vi "Database.vi"(8 "error in (no error)":errorcluster) -> (0 "error out":errorcluster)   [LabVIEW 2017]
uses:
  Type Definitions/Queue FG Options.ctl
  Type Definitions/DB Data.ctl
  Type Definitions/DB Info.ctl
  Type Definitions/Controller Message.ctl
  Type Definitions/Controller States.ctl
  Type Definitions/Controller Data.ctl
  Type Definitions/Display Data.ctl
  Type Definitions/DB Record.ctl
  Type Definitions/Display Console States.ctl
  Type Definitions/GUI Data.ctl
  Type Definitions/Sensor UI Data.ctl
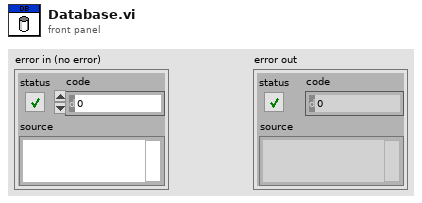
[diagram p1: front panel]
types:
  T1 = typedef "Queue FG Options.ctl" = enum16{"Set", "Get", "Read", "Write", "Destroy"}
  T2 = typedef "DB Data.ctl" = cluster{"Account":i32, "First Name":string, "Last Name":string, "Balance":fxp<+/-,64,35>, "DB Info":T3}
  T3 = typedef "DB Info.ctl" = enum16{"Empty", "Verify", "Login Accepted", "Invalid Login", "Deposit Complete", "Withdrawal Complete", "Withdrawal Failed", "Terminate"}
  T4 = typedef "Controller States.ctl" = enum16{"Timeout", "Initial", "Login", "Idle", "Balance Inquiry", "Deposit", "Withdrawal", "Fast Cash", "Terminate", "Wait on Exit", "Shutdown", "Error Handler"}
  T5 = typedef "Controller Data.ctl" = cluster{"Time":dbl, "DB Data in":T2, "Display Data":T6, "GUI Data ":T9, "Sensor UI":T10, "Controller States":T4}
  T6 = typedef "Display Data.ctl" = cluster{"Message Text":string, "DB Record":T7, "Card Read":bool, "Display Console States":T8}
  T7 = typedef "DB Record.ctl" = cluster{"Account":i32, "First Name":string, "Last Name":string, "Balance":fxp<+/-,64,35>}
  T8 = typedef "Display Console States.ctl" = enum16{"Timeout", "Initial", "Login", "Invalid Login", "Idle", "Balance Inquiry", "Deposit", "Withdrawal", "Fast Cash", "Withdrawal Failed", "Withdrawal Complete", "Terminate", "Shutdown"}
  T9 = typedef "GUI Data.ctl" = cluster{"Card Reader":enum8{"Enabled", "Disabled", "Disabled and Grayed Out"}, "Keypad":enum8{"Enabled", "Disabled", "Disabled and Grayed Out"}, "Balance Inquiry":enum8{"Enabled", "Disabled", "Disabled and Grayed Out"}, "Deposit":enum8{"Enabled", "Disabled", "Disabled and Grayed Out"}, "Withdrawal":enum8{"Enabled", "Disabled", "Disabled and Grayed Out"}, "Fast Cash":enum8{"Enabled", "Disabled", "Disabled and Grayed Out"}, "New Transaction":enum8{"Enabled", "Disabled", "Disabled and Grayed Out"}, "Terminate Session":enum8{"Enabled", "Disabled", "Disabled and Grayed Out"}, "Pinpad Value":string, "Timeout":i32, "Controller States":T4}
  T10 = typedef "Sensor UI Data.ctl" = cluster{"Funds dispensed":enum16{"Enabled", "Disabled", "Disabled and Grayed Out"}, "Deposit received":enum16{"Enabled", "Disabled", "Disabled and Grayed Out"}, "Timeout":dbl}
  T11 = typedef "Controller Message.ctl" = cluster{"Message Info":T4, "Message Data":variant}
  T12 = typedef "Database Message.ctl" = cluster{"Message Info":T13, "Message Data":variant}
  T13 = typedef "Database States.ctl" = enum16{"Initial", "Verify", "Balance Inquiry", "Deposit", "Withdrawal", "Fast Cash", "Terminate", "Shutdown"}
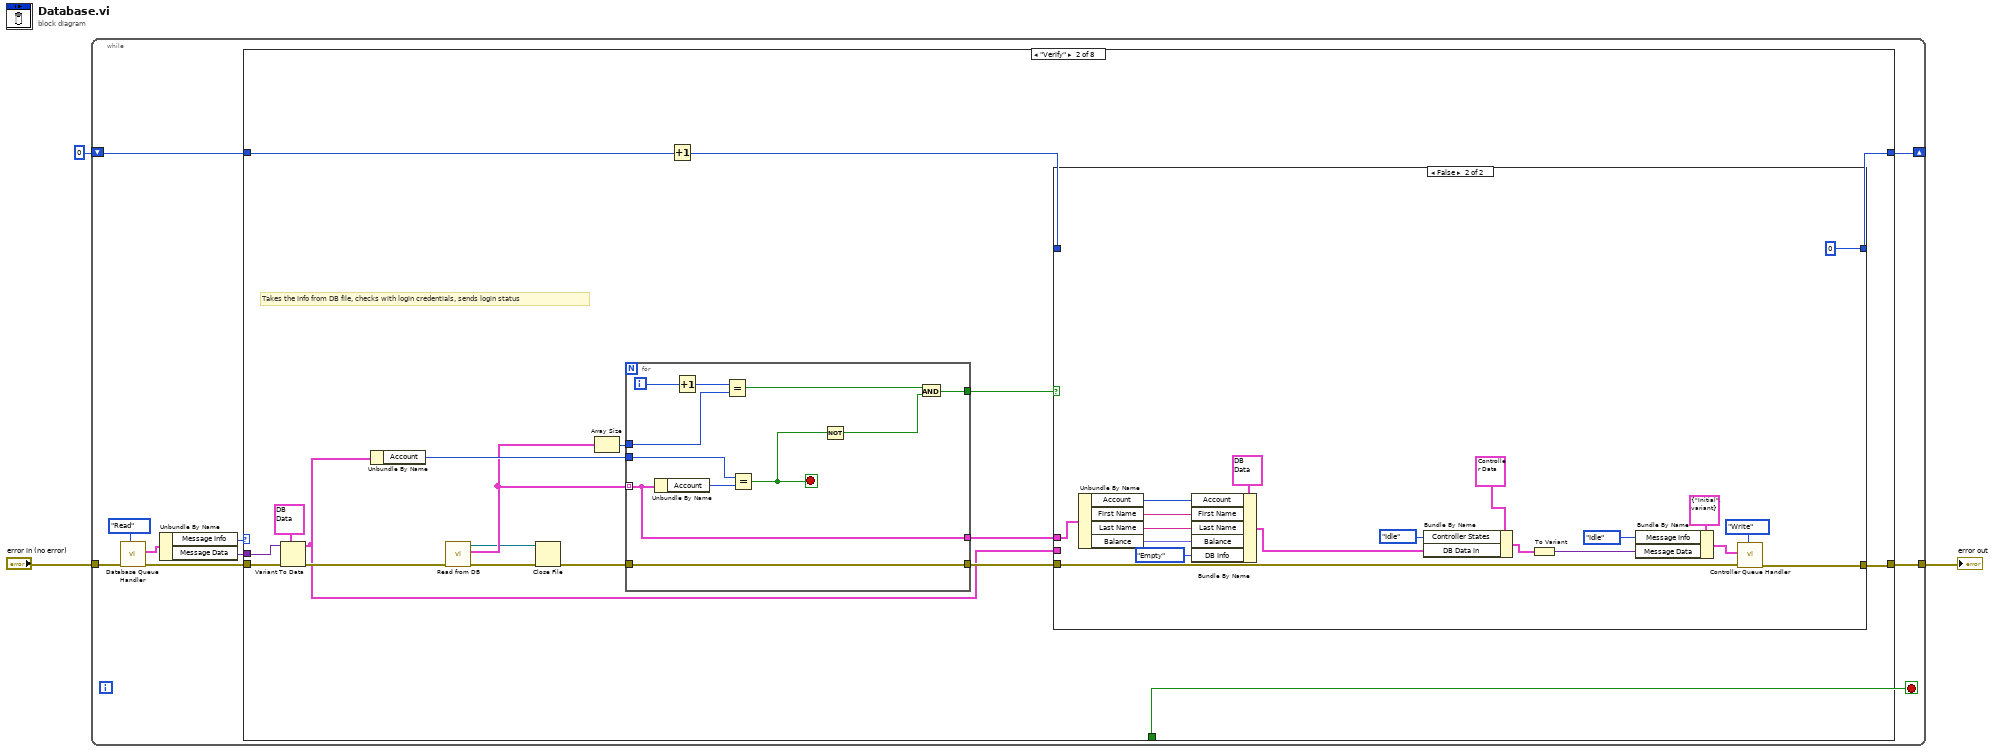
[diagram p0: block diagram]
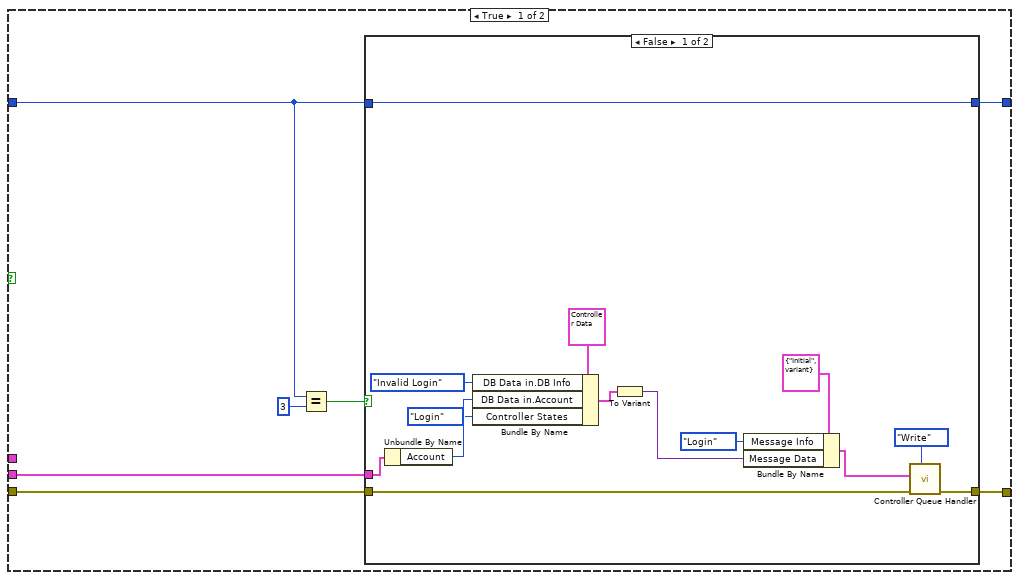
[diagram p3: hidden frame]
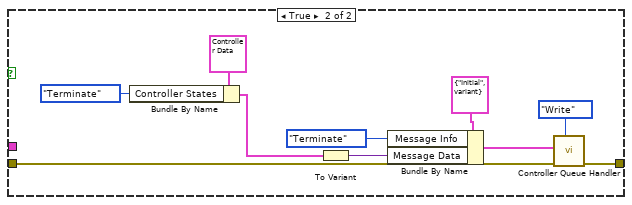
[diagram p4: hidden frame]
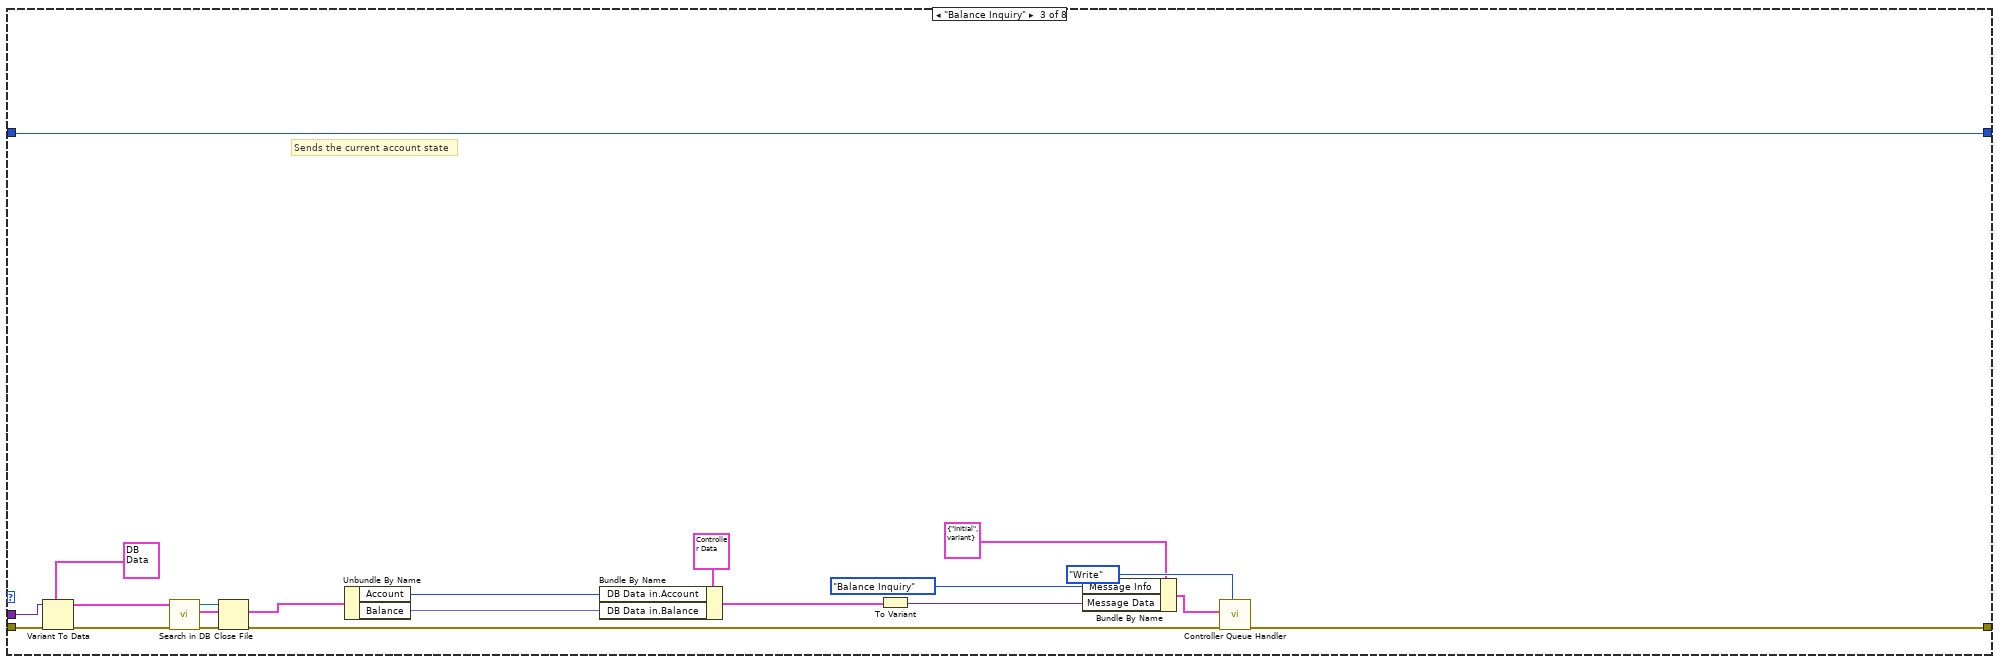
[diagram p5: hidden frame]
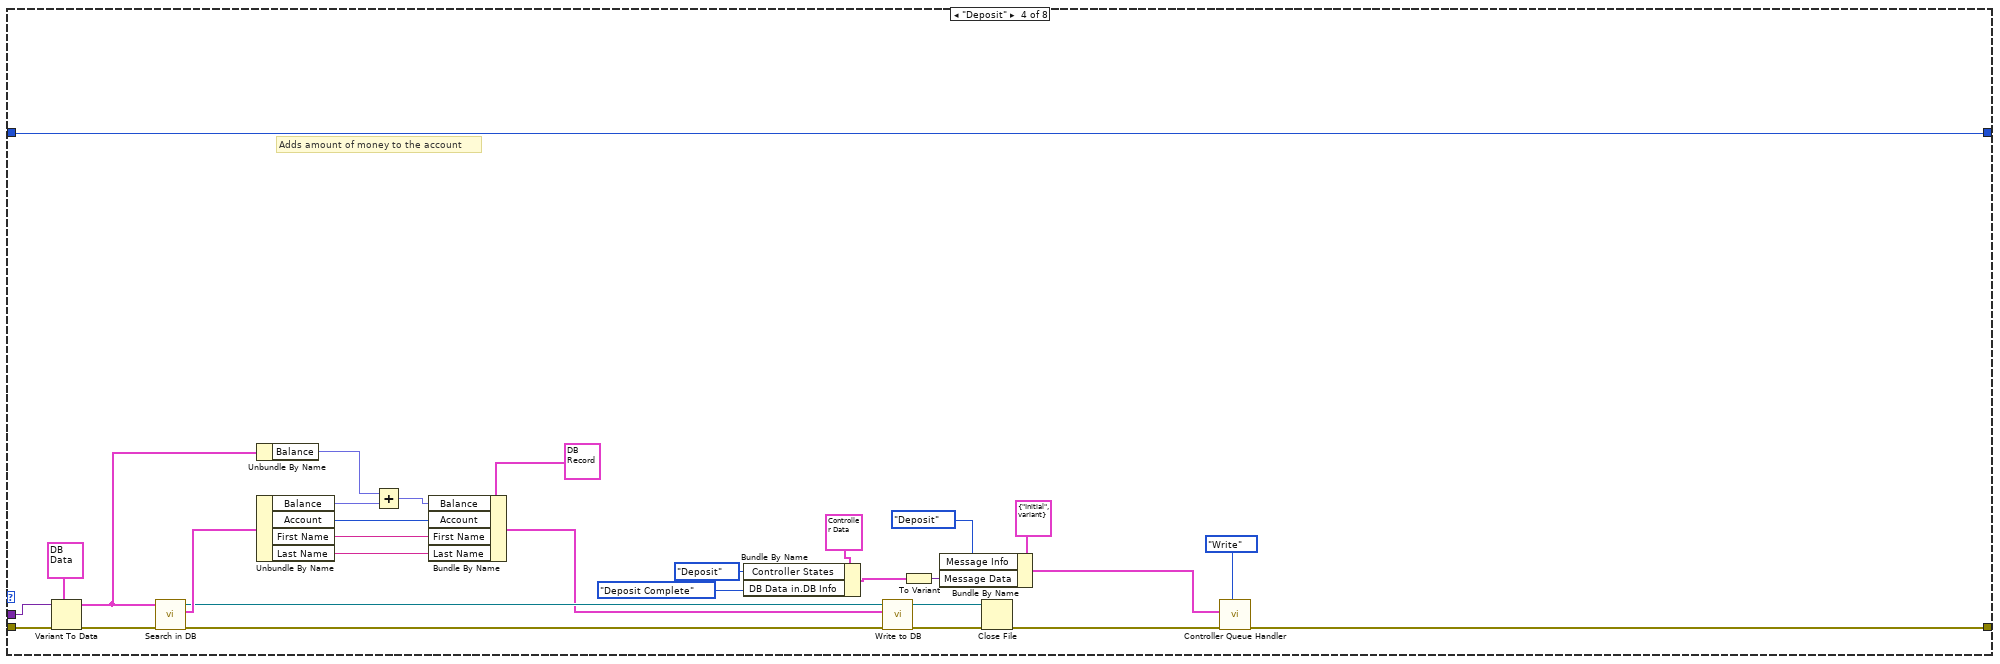
[diagram p6: hidden frame]
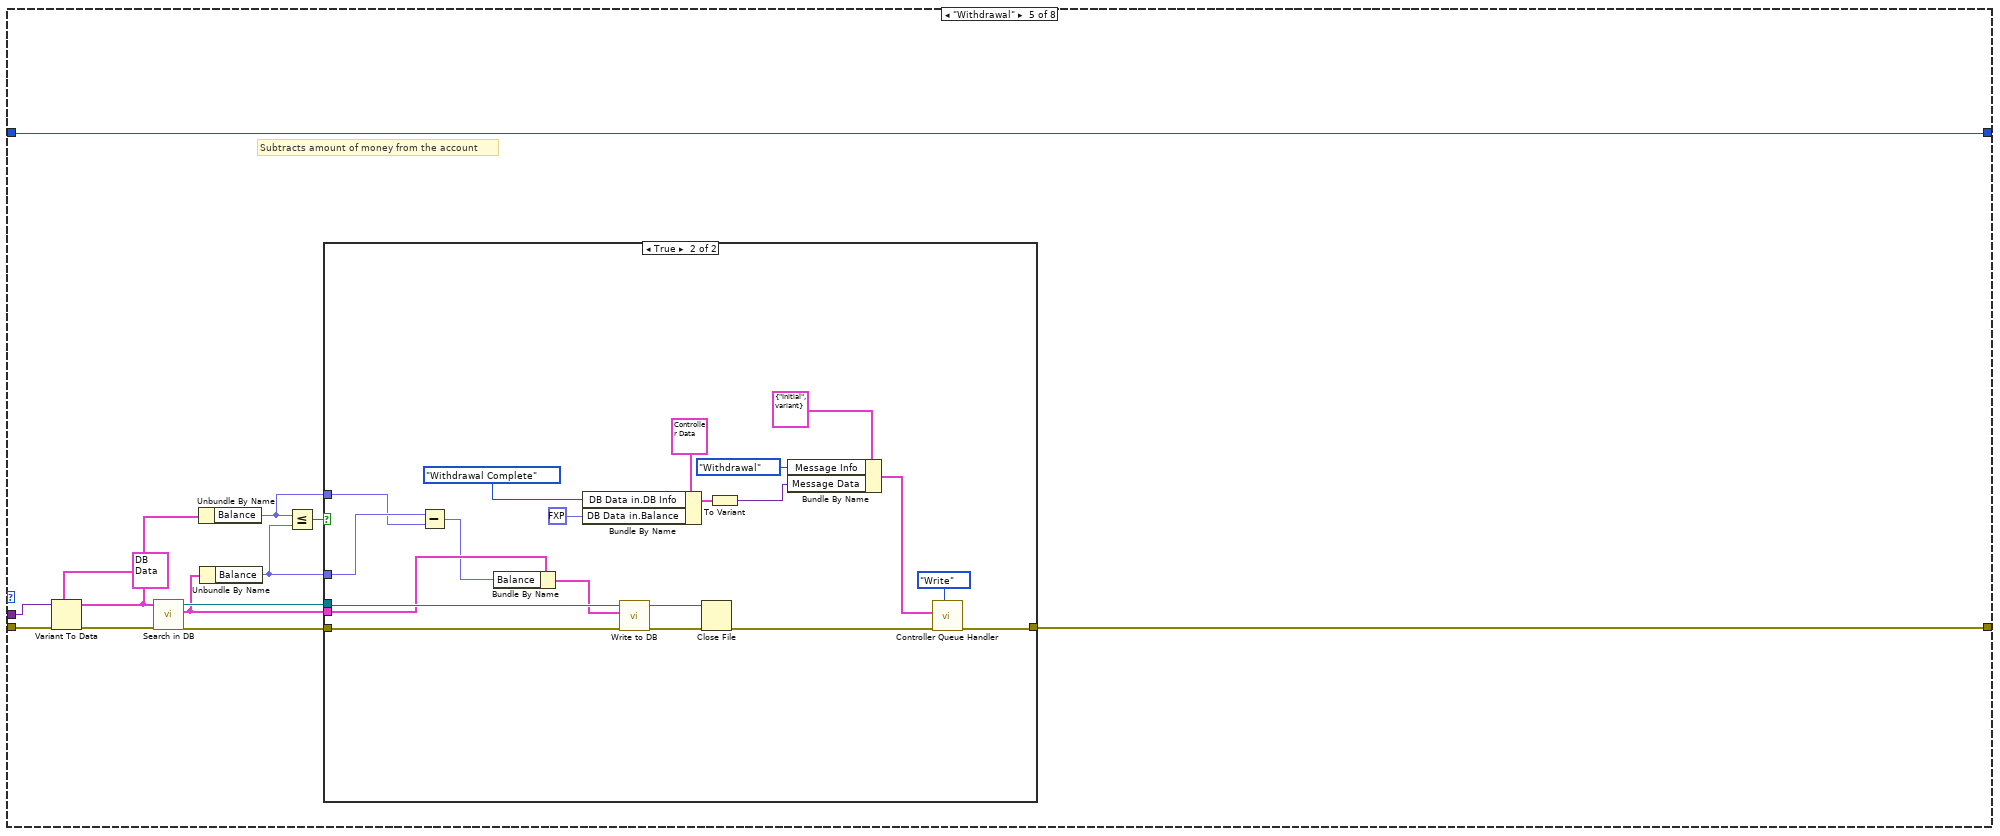
[diagram p7: hidden frame]
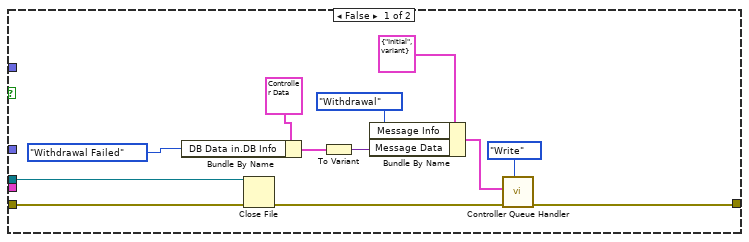
[diagram p8: hidden frame]
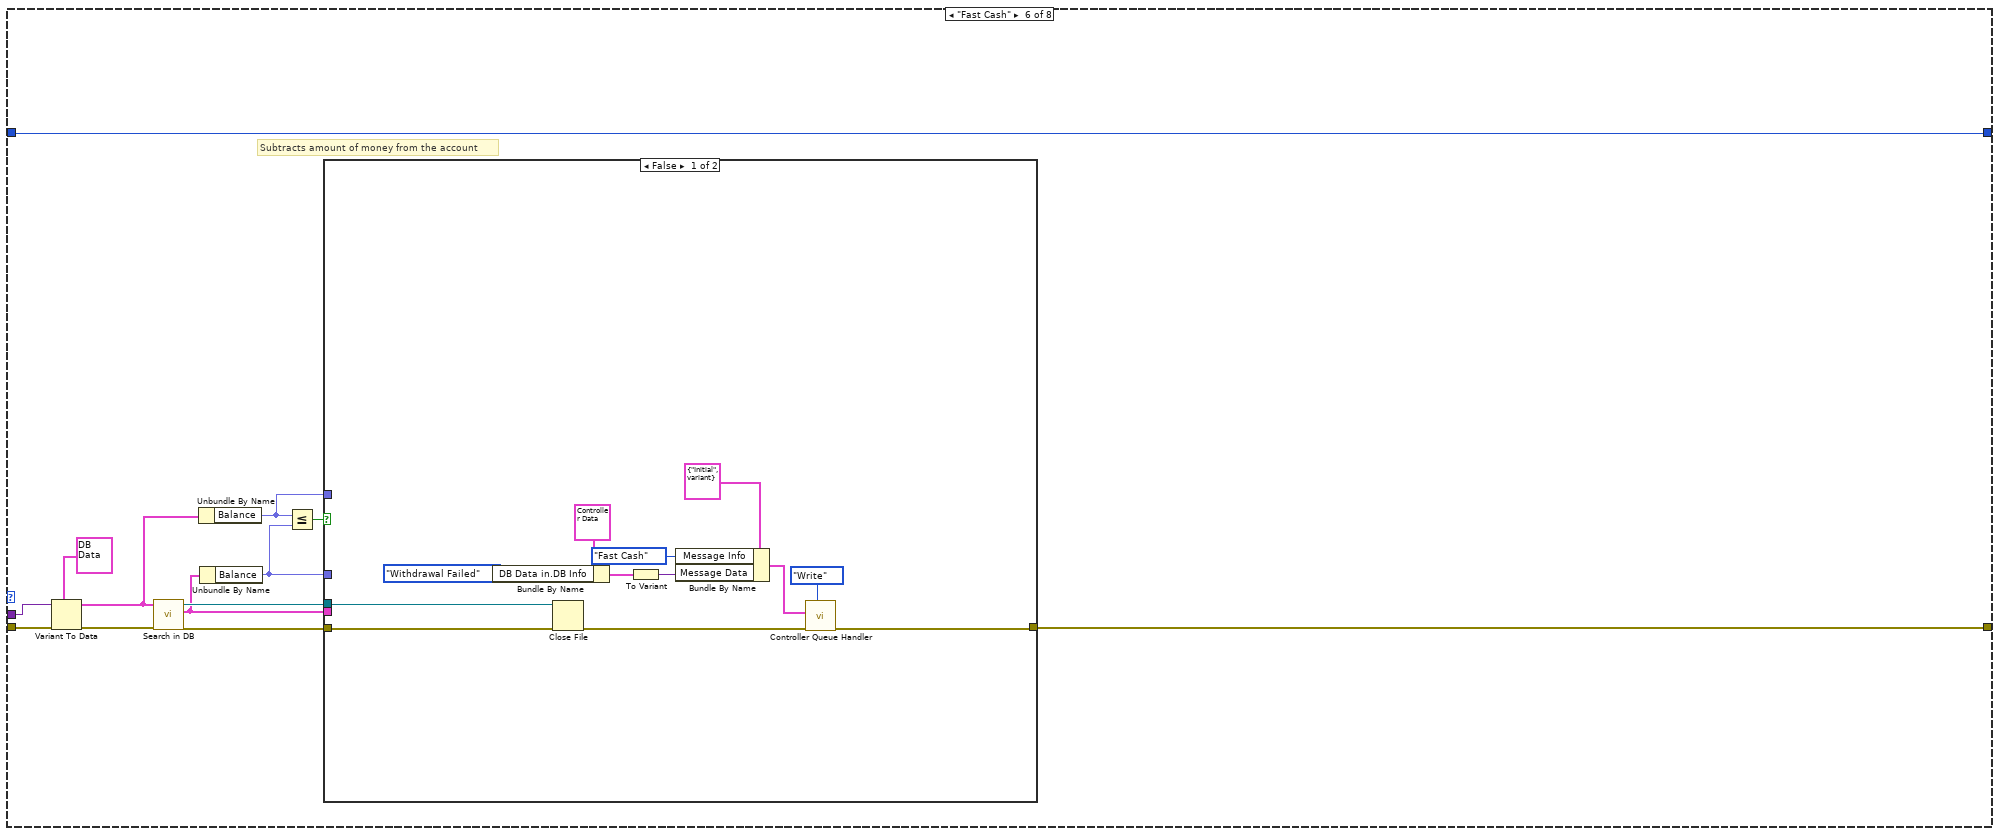
[diagram p9: hidden frame]
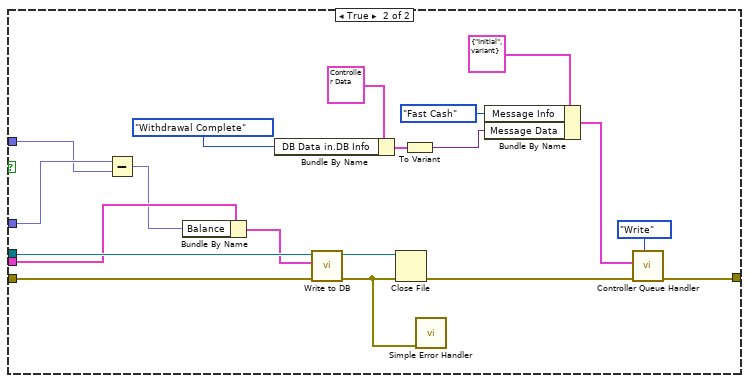
[diagram p10: hidden frame]
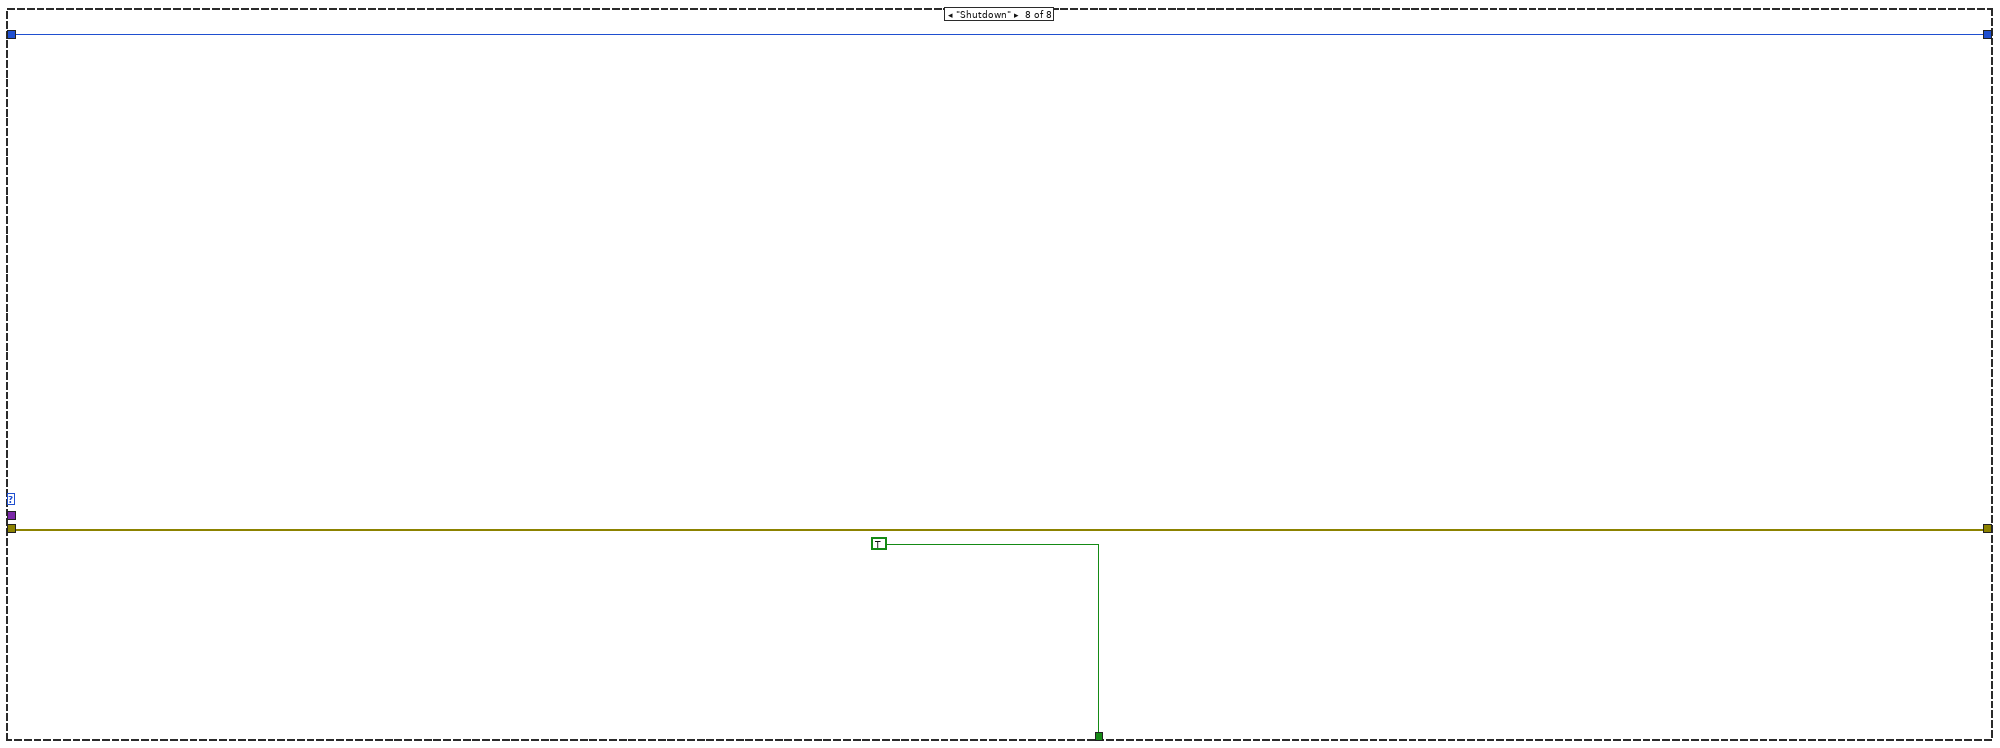
[diagram p12: hidden frame]
diagram:
  n1 = while {
    tunnel: "error in (no error)" -> [w12]
    tunnel: [w7] -> w2
    shift-right: [w5] -> _
    shift-left: 0 -> [w4]
    stop <- w6 stop-if-true
    n2 = call "Database Queue Handler.vi"("Action"=Queue_FG_Options."Read", "error in (no error)"=w12) -> ("error out"=w8:errorcluster, "Message out"=w11:T12)  [unwired: 7 in, 1 out]
    n3 = Unbundle By Name(w11) -> ("Message Info"=w10:T13, "Message Data"=w9:variant)
    n4 = case shown="\"Verify\"" w10 {
      tunnel: w9 -> [_ w31 w111 w141 w154 w199 _ _]
      tunnel: w8 -> [w15 w33 w114 w144 w157 w202 w235 w238]
      tunnel: [w15 w18 w108 w126 w148 w193 w235 w238] -> w7
      tunnel: [_ _ _ _ _ _ _ TRUE] -> w6
      tunnel: [w14 w17 w113 w143 w156 w201 w234 w236] -> w5
      tunnel: w4 -> [w14 w25 w113 w143 w156 w201 w234 w236]
      frame "Initial", Default {
      }
      frame "Verify" {
        # "Takes the info from DB file, checks with login credentials, sends login status"
        n5 = Variant To Data(error in=w33, type=T2 {"Account"=0, "First Name"="", "Last Name"="", "Balance"=0.0, "DB Info"=enum."Login Accepted"} ("DB Data in"), Variant=w31) -> (data=w20:T2, error out=w32:errorcluster)
        n6 = Unbundle By Name(w20) -> ("Account"=w29:i32)
        n7 = call "Read from DB.vi"("error in (no error)"=w32) -> ("error out"=w28:errorcluster, "Array"=w23:T7[], "refnum out"=w21:refnum<file>)  [unwired: 8 in]
        n8 = Close File(refnum=w21, error in=w28) -> (error out=w22:errorcluster)  [unwired: 1 out]
        n9 = Array Size(array=w23) -> (size(s)=w27:i32)
        n10 = for {
          tunnel: w29 -> [w43]
          tunnel: w23 -> [w34] mode=indexing
          tunnel: w22 -> [w35]
          tunnel: [w35] -> w24
          tunnel: w27 -> [w40]
          tunnel: [w36] -> w26
          tunnel: [w34] -> w16
          i -> [w42]
          stop <- w39 stop-if-true
          n11 = Unbundle By Name(w34) -> ("Account"=w44:i32)
          n12 = Increment(x=w42) -> (x+1=w41:i32)
          n13 = Equal?(x=w41, y=w40) -> (x = y?=w37:bool)
          n14 = Equal?(x=w43, y=w44) -> (x = y?=w39:bool)
          n15 = Not(x=w39) -> (.not. x?=w38:bool)
          n16 = And(x=w37, y=w38) -> (x .and. y?=w36:bool)
        }
        n17 = Increment(x=w25) -> (x+1=w19:i32)
        n18 = case shown="False" w26 {
          tunnel: w19 -> [w51 _]
          tunnel: w24 -> [w50 w86]
          tunnel: w20 -> [w47 _]
          tunnel: [w45 w85] -> w18
          tunnel: [w46 0] -> w17
          tunnel: w16 -> [_ w81]
          frame True {
            n19 = Equal?(x=w51, y=3) -> (x = y?=w48:bool)
            n20 = case shown="False" w48 {
              tunnel: w50 -> [w65 w75]
              tunnel: [w64 w74] -> w45
              tunnel: w51 -> [w56 _]
              tunnel: [w56 _] -> w46
              tunnel: w47 -> [w53 _]
              frame False {
                n21 = Unbundle By Name(w53) -> ("Account"=w54:i32)
                n22 = Bundle By Name(cluster=T5 {"Time"=0.0, "DB Data in"={"Account"=0, "First Name"="", "Last Name"="", "Balance"=0.0, "DB Info"=enum."Login Accepted"}, "Display Data"={"Message Text"="", "DB Record"={"Account"=0, "First Name"="", "Last Name"="", "Balance"=0.0}, "Card Read"=FALSE, "Display Console States"=enum."Timeout"}, "GUI Data "={"Card Reader"=enum."Enabled", "Keypad"=enum."Enabled", "Balance Inquiry"=enum."Enabled", "Deposit"=enum."Enabled", "Withdrawal"=enum."Enabled", "Fast Cash"=enum."Enabled", "New Transaction"=enum."Enabled", "Terminate Session"=enum."Enabled", "Pinpad Value"="", "Timeout"=0, "Controller States"=enum."Initial"}, "Sensor UI"={"Funds dispensed"=enum."Enabled", "Deposit received"=enum."Enabled", "Timeout"=0.0}, "Controller States"=enum."Timeout"} ("Controller Data"), "DB Data in.DB Info"=DB_Info."Invalid Login" ("DB Info"), "DB Data in.Account"=w54, "Controller States"=Controller_States."Login") -> (w58:T5)
                n23 = To Variant(anything=w58) -> (Variant=w57:variant)
                n24 = Bundle By Name(cluster=T11 {"Message Info"=enum."Initial", "Message Data"=variant} ("Message"), "Message Info"=Controller_States."Login" ("Controller States"), "Message Data"=w57) -> (w60:T11)
                n25 = call "Controller Queue Handler.vi"("Action"=Queue_FG_Options."Write", "error in (no error)"=w65, "Message in"=w60) -> ("error out"=w64:errorcluster)  [unwired: 6 in, 2 out]
              }
              frame True {
                n26 = Bundle By Name(cluster=T5 {"Time"=0.0, "DB Data in"={"Account"=0, "First Name"="", "Last Name"="", "Balance"=0.0, "DB Info"=enum."Login Accepted"}, "Display Data"={"Message Text"="", "DB Record"={"Account"=0, "First Name"="", "Last Name"="", "Balance"=0.0}, "Card Read"=FALSE, "Display Console States"=enum."Timeout"}, "GUI Data "={"Card Reader"=enum."Enabled", "Keypad"=enum."Enabled", "Balance Inquiry"=enum."Enabled", "Deposit"=enum."Enabled", "Withdrawal"=enum."Enabled", "Fast Cash"=enum."Enabled", "New Transaction"=enum."Enabled", "Terminate Session"=enum."Enabled", "Pinpad Value"="", "Timeout"=0, "Controller States"=enum."Initial"}, "Sensor UI"={"Funds dispensed"=enum."Enabled", "Deposit received"=enum."Enabled", "Timeout"=0.0}, "Controller States"=enum."Timeout"} ("Controller Data"), "Controller States"=Controller_States."Terminate") -> (w67:T5)
                n27 = To Variant(anything=w67) -> (Variant=w66:variant)
                n28 = Bundle By Name(cluster=T11 {"Message Info"=enum."Initial", "Message Data"=variant} ("Message"), "Message Info"=Controller_States."Terminate" ("Controller States"), "Message Data"=w66) -> (w70:T11)
                n29 = call "Controller Queue Handler.vi"("Action"=Queue_FG_Options."Write", "error in (no error)"=w75, "Message in"=w70) -> ("error out"=w74:errorcluster)  [unwired: 6 in, 2 out]
              }
            }
          }
          frame False {
            n30 = Unbundle By Name(w81) -> ("Account"=w80:i32, "First Name"=w79:string, "Last Name"=w78:string, "Balance"=w77:fxp<+/-,64,35>)
            n31 = Bundle By Name(cluster=T2 {"Account"=0, "First Name"="", "Last Name"="", "Balance"=0.0, "DB Info"=enum."Login Accepted"} ("DB Data in"), "Account"=w80, "First Name"=w79, "Last Name"=w78, "Balance"=w77, "DB Info"=DB_Info."Empty") -> (w82:T2)
            n32 = Bundle By Name(cluster=T5 {"Time"=0.0, "DB Data in"={"Account"=0, "First Name"="", "Last Name"="", "Balance"=0.0, "DB Info"=enum."Login Accepted"}, "Display Data"={"Message Text"="", "DB Record"={"Account"=0, "First Name"="", "Last Name"="", "Balance"=0.0}, "Card Read"=FALSE, "Display Console States"=enum."Timeout"}, "GUI Data "={"Card Reader"=enum."Enabled", "Keypad"=enum."Enabled", "Balance Inquiry"=enum."Enabled", "Deposit"=enum."Enabled", "Withdrawal"=enum."Enabled", "Fast Cash"=enum."Enabled", "New Transaction"=enum."Enabled", "Terminate Session"=enum."Enabled", "Pinpad Value"="", "Timeout"=0, "Controller States"=enum."Initial"}, "Sensor UI"={"Funds dispensed"=enum."Enabled", "Deposit received"=enum."Enabled", "Timeout"=0.0}, "Controller States"=enum."Timeout"} ("Controller Data"), "Controller States"=Controller_States."Idle", "DB Data in"=w82) -> (w90:T5)
            n33 = To Variant(anything=w90) -> (Variant=w89:variant)
            n34 = Bundle By Name(cluster=T11 {"Message Info"=enum."Initial", "Message Data"=variant} ("Message"), "Message Info"=Controller_States."Idle", "Message Data"=w89) -> (w93:T11)
            n35 = call "Controller Queue Handler.vi"("Action"=Queue_FG_Options."Write", "error in (no error)"=w86, "Message in"=w93) -> ("error out"=w85:errorcluster)  [unwired: 6 in, 2 out]
          }
        }
      }
      frame "Balance Inquiry" {
        # "Sends the current account state"
        n36 = Variant To Data(error in=w114, type=T2 {"Account"=0, "First Name"="", "Last Name"="", "Balance"=0.0, "DB Info"=enum."Login Accepted"} ("DB Data in"), Variant=w111) -> (data=w109:T2, error out=w112:errorcluster)
        n37 = call "Search in DB.vi"("error in (no error)"=w112, "DB Data in"=w109) -> ("error out"=w96:errorcluster, "DB Record"=w100:T7, "refnum out"=w97:refnum<file>)  [unwired: 7 in]
        n38 = Close File(refnum=w97, error in=w96) -> (error out=w95:errorcluster)  [unwired: 1 out]
        n39 = Unbundle By Name(w100) -> ("Account"=w99:i32, "Balance"=w98:fxp<+/-,64,35>)
        n40 = Bundle By Name(cluster=T5 {"Time"=0.0, "DB Data in"={"Account"=0, "First Name"="", "Last Name"="", "Balance"=0.0, "DB Info"=enum."Login Accepted"}, "Display Data"={"Message Text"="", "DB Record"={"Account"=0, "First Name"="", "Last Name"="", "Balance"=0.0}, "Card Read"=FALSE, "Display Console States"=enum."Timeout"}, "GUI Data "={"Card Reader"=enum."Enabled", "Keypad"=enum."Enabled", "Balance Inquiry"=enum."Enabled", "Deposit"=enum."Enabled", "Withdrawal"=enum."Enabled", "Fast Cash"=enum."Enabled", "New Transaction"=enum."Enabled", "Terminate Session"=enum."Enabled", "Pinpad Value"="", "Timeout"=0, "Controller States"=enum."Initial"}, "Sensor UI"={"Funds dispensed"=enum."Enabled", "Deposit received"=enum."Enabled", "Timeout"=0.0}, "Controller States"=enum."Timeout"} ("Controller Data"), "DB Data in.Account"=w99, "DB Data in.Balance"=w98) -> (w105:T5)
        n41 = To Variant(anything=w105) -> (Variant=w103:variant)
        n42 = Bundle By Name(cluster=T11 {"Message Info"=enum."Initial", "Message Data"=variant} ("Message"), "Message Info"=Controller_States."Balance Inquiry", "Message Data"=w103) -> (w101:T11)
        n43 = call "Controller Queue Handler.vi"("Action"=Queue_FG_Options."Write", "error in (no error)"=w95, "Message in"=w101) -> ("error out"=w108:errorcluster)  [unwired: 6 in, 2 out]
      }
      frame "Deposit" {
        # "Adds amount of money to the account"
        n44 = Variant To Data(error in=w144, type=T2 {"Account"=0, "First Name"="", "Last Name"="", "Balance"=0.0, "DB Info"=enum."Login Accepted"} ("DB Data in"), Variant=w141) -> (data=w138:T2, error out=w142:errorcluster)
        n45 = call "Search in DB.vi"("error in (no error)"=w142, "DB Data in"=w138) -> ("error out"=w139:errorcluster, "DB Record"=w130:T7, "refnum out"=w128:refnum<file>)  [unwired: 7 in]
        n46 = Unbundle By Name(w138) -> ("Balance"=w132:fxp<+/-,64,35>)
        n47 = Unbundle By Name(w130) -> ("Balance"=w133:fxp<+/-,64,35>, "Account"=w136:i32, "First Name"=w135:string, "Last Name"=w134:string)
        n48 = Add(x=w132, y=w133) -> (x+y=w131:fxp<+/-,64,36>)
        n49 = Bundle By Name(cluster=T7 {"Account"=0, "First Name"="", "Last Name"="", "Balance"=0.0} ("DB Record"), "Balance"=w131, "Account"=w136, "First Name"=w135, "Last Name"=w134) -> (w127:T7)
        n50 = Bundle By Name(cluster=T5 {"Time"=0.0, "DB Data in"={"Account"=0, "First Name"="", "Last Name"="", "Balance"=0.0, "DB Info"=enum."Login Accepted"}, "Display Data"={"Message Text"="", "DB Record"={"Account"=0, "First Name"="", "Last Name"="", "Balance"=0.0}, "Card Read"=FALSE, "Display Console States"=enum."Timeout"}, "GUI Data "={"Card Reader"=enum."Enabled", "Keypad"=enum."Enabled", "Balance Inquiry"=enum."Enabled", "Deposit"=enum."Enabled", "Withdrawal"=enum."Enabled", "Fast Cash"=enum."Enabled", "New Transaction"=enum."Enabled", "Terminate Session"=enum."Enabled", "Pinpad Value"="", "Timeout"=0, "Controller States"=enum."Initial"}, "Sensor UI"={"Funds dispensed"=enum."Enabled", "Deposit received"=enum."Enabled", "Timeout"=0.0}, "Controller States"=enum."Timeout"} ("Controller Data"), "Controller States"=Controller_States."Deposit", "DB Data in.DB Info"=DB_Info."Deposit Complete") -> (w117:T5)
        n51 = call "Write to DB.vi"("error in (no error)"=w139, "DB Record"=w127, "refnum"=w128) -> ("error out"=w129:errorcluster, "refnum out"=w123:refnum<file>)  [unwired: 7 in]
        n52 = To Variant(anything=w117) -> (Variant=w116:variant)
        n53 = Bundle By Name(cluster=T11 {"Message Info"=enum."Initial", "Message Data"=variant} ("Message"), "Message Info"=Controller_States."Deposit", "Message Data"=w116) -> (w120:T11)
        n54 = Close File(refnum=w123, error in=w129) -> (error out=w124:errorcluster)  [unwired: 1 out]
        n55 = call "Controller Queue Handler.vi"("Action"=Queue_FG_Options."Write", "error in (no error)"=w124, "Message in"=w120) -> ("error out"=w126:errorcluster)  [unwired: 6 in, 2 out]
      }
      frame "Withdrawal" {
        # "Subtracts amount of money from the account"
        n56 = Variant To Data(error in=w157, type=T2 {"Account"=0, "First Name"="", "Last Name"="", "Balance"=0.0, "DB Info"=enum."Login Accepted"} ("DB Data in"), Variant=w154) -> (data=w152:T2, error out=w155:errorcluster)
        n57 = call "Search in DB.vi"("error in (no error)"=w155, "DB Data in"=w152) -> ("error out"=w149:errorcluster, "DB Record"=w145:T7, "refnum out"=w150:refnum<file>)  [unwired: 7 in]
        n58 = Unbundle By Name(w152) -> ("Balance"=w147:fxp<+/-,64,35>)
        n59 = Unbundle By Name(w145) -> ("Balance"=w146:fxp<+/-,64,35>)
        n60 = Less Or Equal?(x=w147, y=w146) -> (x <= y?=w151:bool)
        n61 = case shown="True" w151 {
          tunnel: w150 -> [w158 w188]
          tunnel: w149 -> [w169 w189]
          tunnel: [w168 w179] -> w148
          tunnel: w147 -> [_ w186]
          tunnel: w146 -> [_ w187]
          tunnel: w145 -> [_ w185]
          frame False {
            n62 = Bundle By Name(cluster=T5 {"Time"=0.0, "DB Data in"={"Account"=0, "First Name"="", "Last Name"="", "Balance"=0.0, "DB Info"=enum."Login Accepted"}, "Display Data"={"Message Text"="", "DB Record"={"Account"=0, "First Name"="", "Last Name"="", "Balance"=0.0}, "Card Read"=FALSE, "Display Console States"=enum."Timeout"}, "GUI Data "={"Card Reader"=enum."Enabled", "Keypad"=enum."Enabled", "Balance Inquiry"=enum."Enabled", "Deposit"=enum."Enabled", "Withdrawal"=enum."Enabled", "Fast Cash"=enum."Enabled", "New Transaction"=enum."Enabled", "Terminate Session"=enum."Enabled", "Pinpad Value"="", "Timeout"=0, "Controller States"=enum."Initial"}, "Sensor UI"={"Funds dispensed"=enum."Enabled", "Deposit received"=enum."Enabled", "Timeout"=0.0}, "Controller States"=enum."Timeout"} ("Controller Data"), "DB Data in.DB Info"=DB_Info."Withdrawal Failed" ("DB Info")) -> (w161:T5)
            n63 = Close File(refnum=w158, error in=w169) -> (error out=w159:errorcluster)  [unwired: 1 out]
            n64 = To Variant(anything=w161) -> (Variant=w160:variant)
            n65 = Bundle By Name(cluster=T11 {"Message Info"=enum."Initial", "Message Data"=variant} ("Message"), "Message Info"=Controller_States."Withdrawal", "Message Data"=w160) -> (w166:T11)
            n66 = call "Controller Queue Handler.vi"("Action"=Queue_FG_Options."Write", "error in (no error)"=w159, "Message in"=w166) -> ("error out"=w168:errorcluster)  [unwired: 6 in, 2 out]
          }
          frame True {
            n67 = Subtract(x=w187, y=w186) -> (x-y=w184:fxp<+/-,64,36>)
            n68 = Bundle By Name(cluster=w185, "Balance"=w184) -> (w183:T7)
            n69 = Bundle By Name(cluster=T5 {"Time"=0.0, "DB Data in"={"Account"=0, "First Name"="", "Last Name"="", "Balance"=0.0, "DB Info"=enum."Login Accepted"}, "Display Data"={"Message Text"="", "DB Record"={"Account"=0, "First Name"="", "Last Name"="", "Balance"=0.0}, "Card Read"=FALSE, "Display Console States"=enum."Timeout"}, "GUI Data "={"Card Reader"=enum."Enabled", "Keypad"=enum."Enabled", "Balance Inquiry"=enum."Enabled", "Deposit"=enum."Enabled", "Withdrawal"=enum."Enabled", "Fast Cash"=enum."Enabled", "New Transaction"=enum."Enabled", "Terminate Session"=enum."Enabled", "Pinpad Value"="", "Timeout"=0, "Controller States"=enum."Initial"}, "Sensor UI"={"Funds dispensed"=enum."Enabled", "Deposit received"=enum."Enabled", "Timeout"=0.0}, "Controller States"=enum."Timeout"} ("Controller Data"), "DB Data in.DB Info"=DB_Info."Withdrawal Complete" ("DB Info"), "DB Data in.Balance"=fxp<+/-,64,35> 0.0 ("Balance")) -> (w173:T5)
            n70 = call "Write to DB.vi"("error in (no error)"=w189, "DB Record"=w183, "refnum"=w188) -> ("error out"=w182:errorcluster, "refnum out"=w180:refnum<file>)  [unwired: 7 in]
            n71 = Close File(refnum=w180, error in=w182) -> (error out=w181:errorcluster)  [unwired: 1 out]
            n72 = To Variant(anything=w173) -> (Variant=w172:variant)
            n73 = Bundle By Name(cluster=T11 {"Message Info"=enum."Initial", "Message Data"=variant} ("Message"), "Message Info"=Controller_States."Withdrawal", "Message Data"=w172) -> (w176:T11)
            n74 = call "Controller Queue Handler.vi"("Action"=Queue_FG_Options."Write", "error in (no error)"=w181, "Message in"=w176) -> ("error out"=w179:errorcluster)  [unwired: 6 in, 2 out]
          }
        }
      }
      frame "Fast Cash" {
        # "Subtracts amount of money from the account"
        n75 = Variant To Data(error in=w202, type=T2 {"Account"=0, "First Name"="", "Last Name"="", "Balance"=0.0, "DB Info"=enum."Login Accepted"} ("DB Data in"), Variant=w199) -> (data=w197:T2, error out=w200:errorcluster)
        n76 = call "Search in DB.vi"("error in (no error)"=w200, "DB Data in"=w197) -> ("error out"=w194:errorcluster, "DB Record"=w190:T7, "refnum out"=w195:refnum<file>)  [unwired: 7 in]
        n77 = Unbundle By Name(w197) -> ("Balance"=w192:fxp<+/-,64,35>)
        n78 = Unbundle By Name(w190) -> ("Balance"=w191:fxp<+/-,64,35>)
        n79 = Less Or Equal?(x=w192, y=w191) -> (x <= y?=w196:bool)
        n80 = case shown="False" w196 {
          tunnel: w195 -> [w203 w232]
          tunnel: w194 -> [w214 w233]
          tunnel: [w213 w224] -> w193
          tunnel: w192 -> [_ w230]
          tunnel: w191 -> [_ w231]
          tunnel: w190 -> [_ w229]
          frame False {
            n81 = Bundle By Name(cluster=T5 {"Time"=0.0, "DB Data in"={"Account"=0, "First Name"="", "Last Name"="", "Balance"=0.0, "DB Info"=enum."Login Accepted"}, "Display Data"={"Message Text"="", "DB Record"={"Account"=0, "First Name"="", "Last Name"="", "Balance"=0.0}, "Card Read"=FALSE, "Display Console States"=enum."Timeout"}, "GUI Data "={"Card Reader"=enum."Enabled", "Keypad"=enum."Enabled", "Balance Inquiry"=enum."Enabled", "Deposit"=enum."Enabled", "Withdrawal"=enum."Enabled", "Fast Cash"=enum."Enabled", "New Transaction"=enum."Enabled", "Terminate Session"=enum."Enabled", "Pinpad Value"="", "Timeout"=0, "Controller States"=enum."Initial"}, "Sensor UI"={"Funds dispensed"=enum."Enabled", "Deposit received"=enum."Enabled", "Timeout"=0.0}, "Controller States"=enum."Timeout"} ("Controller Data"), "DB Data in.DB Info"=DB_Info."Withdrawal Failed" ("DB Info")) -> (w206:T5)
            n82 = Close File(refnum=w203, error in=w214) -> (error out=w204:errorcluster)  [unwired: 1 out]
            n83 = To Variant(anything=w206) -> (Variant=w205:variant)
            n84 = Bundle By Name(cluster=T11 {"Message Info"=enum."Initial", "Message Data"=variant} ("Message"), "Message Info"=Controller_States."Fast Cash", "Message Data"=w205) -> (w211:T11)
            n85 = call "Controller Queue Handler.vi"("Action"=Queue_FG_Options."Write", "error in (no error)"=w204, "Message in"=w211) -> ("error out"=w213:errorcluster)  [unwired: 6 in, 2 out]
          }
          frame True {
            n86 = Subtract(x=w231, y=w230) -> (x-y=w228:fxp<+/-,64,36>)
            n87 = Bundle By Name(cluster=w229, "Balance"=w228) -> (w227:T7)
            n88 = Bundle By Name(cluster=T5 {"Time"=0.0, "DB Data in"={"Account"=0, "First Name"="", "Last Name"="", "Balance"=0.0, "DB Info"=enum."Login Accepted"}, "Display Data"={"Message Text"="", "DB Record"={"Account"=0, "First Name"="", "Last Name"="", "Balance"=0.0}, "Card Read"=FALSE, "Display Console States"=enum."Timeout"}, "GUI Data "={"Card Reader"=enum."Enabled", "Keypad"=enum."Enabled", "Balance Inquiry"=enum."Enabled", "Deposit"=enum."Enabled", "Withdrawal"=enum."Enabled", "Fast Cash"=enum."Enabled", "New Transaction"=enum."Enabled", "Terminate Session"=enum."Enabled", "Pinpad Value"="", "Timeout"=0, "Controller States"=enum."Initial"}, "Sensor UI"={"Funds dispensed"=enum."Enabled", "Deposit received"=enum."Enabled", "Timeout"=0.0}, "Controller States"=enum."Timeout"} ("Controller Data"), "DB Data in.DB Info"=DB_Info."Withdrawal Complete" ("DB Info")) -> (w217:T5)
            n89 = call "Write to DB.vi"("error in (no error)"=w233, "DB Record"=w227, "refnum"=w232) -> ("error out"=w215:errorcluster, "refnum out"=w225:refnum<file>)  [unwired: 7 in]
            n90 = Close File(refnum=w225, error in=w215) -> (error out=w226:errorcluster)  [unwired: 1 out]
            n91 = To Variant(anything=w217) -> (Variant=w216:variant)
            n92 = call <vilib>:"Simple Error Handler.vi"("error in (no error)"=w215) -> ()  [unwired: 4 in, 5 out]
            n93 = Bundle By Name(cluster=T11 {"Message Info"=enum."Initial", "Message Data"=variant} ("Message"), "Message Info"=Controller_States."Fast Cash", "Message Data"=w216) -> (w221:T11)
            n94 = call "Controller Queue Handler.vi"("Action"=Queue_FG_Options."Write", "error in (no error)"=w226, "Message in"=w221) -> ("error out"=w224:errorcluster)  [unwired: 6 in, 2 out]
          }
        }
      }
      frame "Terminate" {
        # "Sends information Terminate to Controller"
      }
      frame "Shutdown" {
      }
    }
  }
  "error out" <- w2
